vi "calc_rot.vi"(3 "Reference":T1, 4 "Input":T3, 5 "img":u8[][](array[numeric])) -> (0 "Close enough":bool, 1 "angle":dbl, 2 "Output":T2)   [LabVIEW 2024]
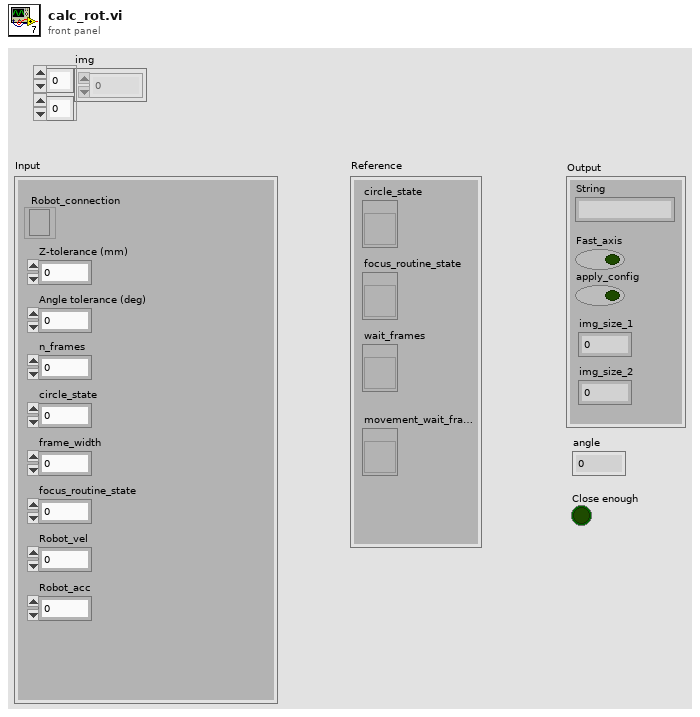
[diagram p1: front panel]
types:
  T1 = cluster{"circle_state":refnum<vi>, "focus_routine_state":refnum<vi>, "wait_frames":refnum<vi>, "movement_wait_frames":refnum<vi>}
  T2 = cluster{"String":string, "Fast_axis":bool, "apply_config":bool, "img_size_1":i32, "img_size_2":i32}
  T3 = cluster{"Robot_connection":refnum<k5>, "Z-tolerance (mm)":dbl, "Angle tolerance (deg)":dbl, "n_frames":i16, "circle_state":i8, "frame_width":i16, "focus_routine_state":i8, "Robot_vel":dbl, "Robot_acc":dbl}
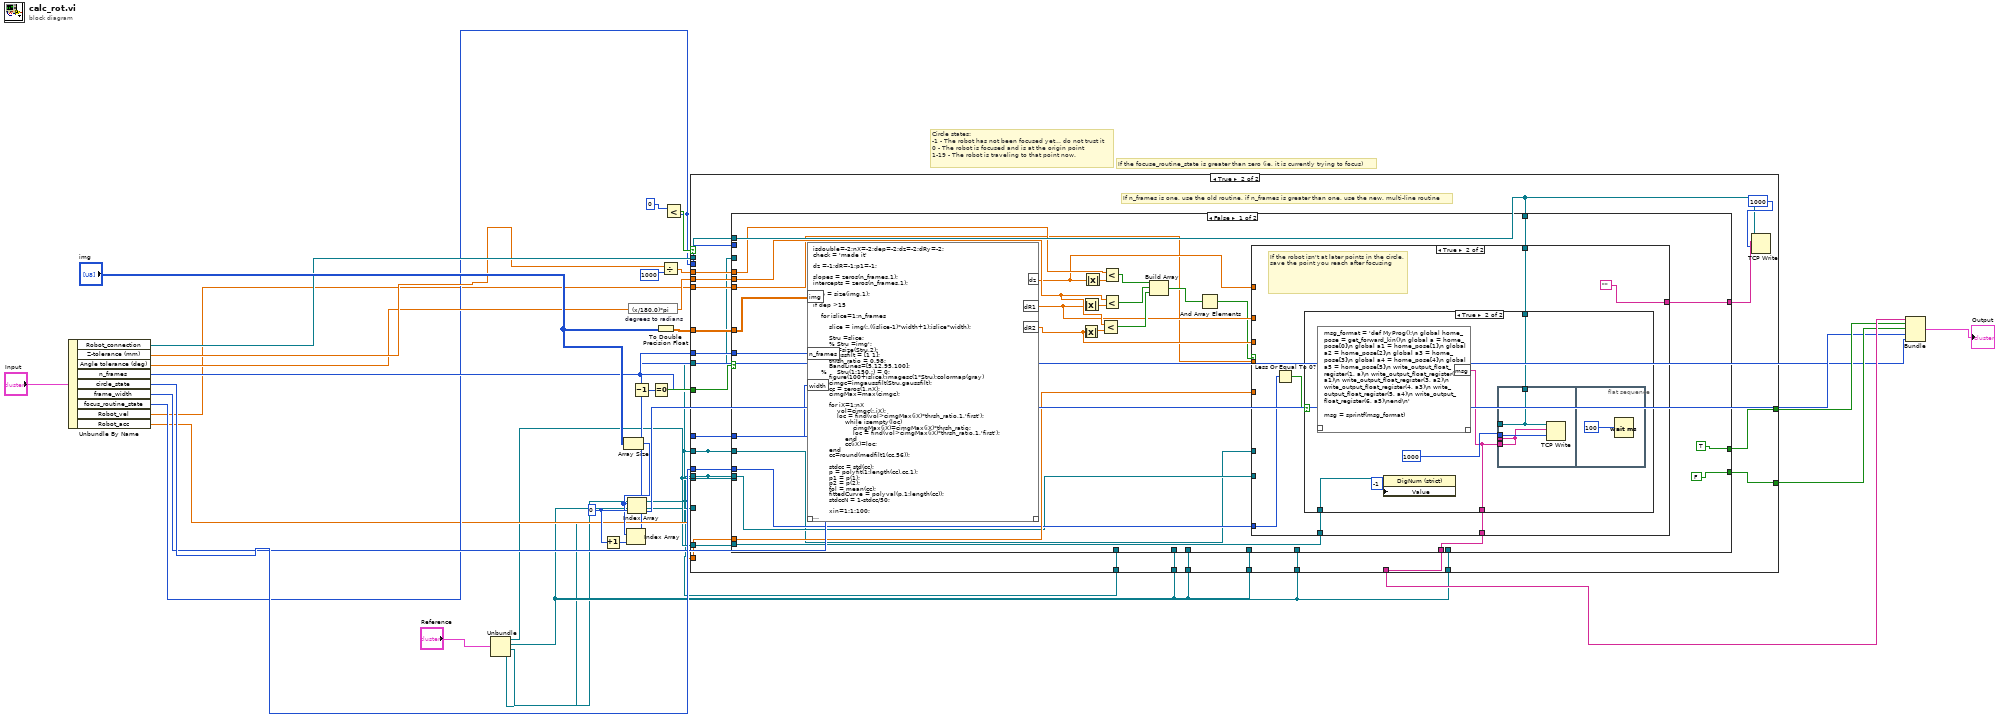
[diagram p0: block diagram]
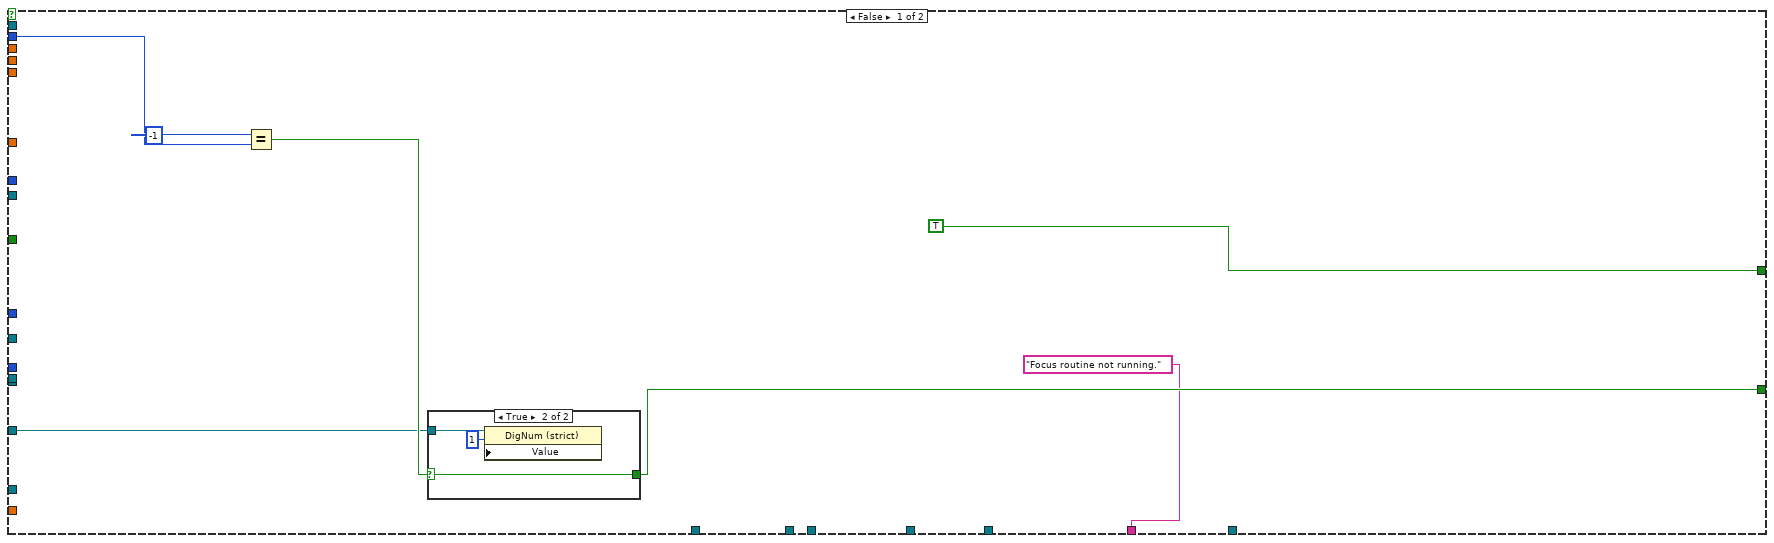
[diagram p2: hidden frame]
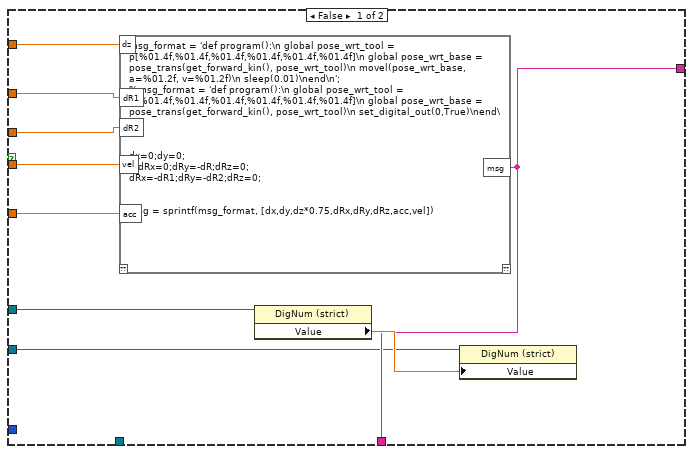
[diagram p4: hidden frame]
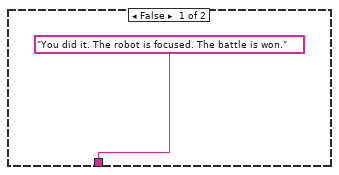
[diagram p5: hidden frame]
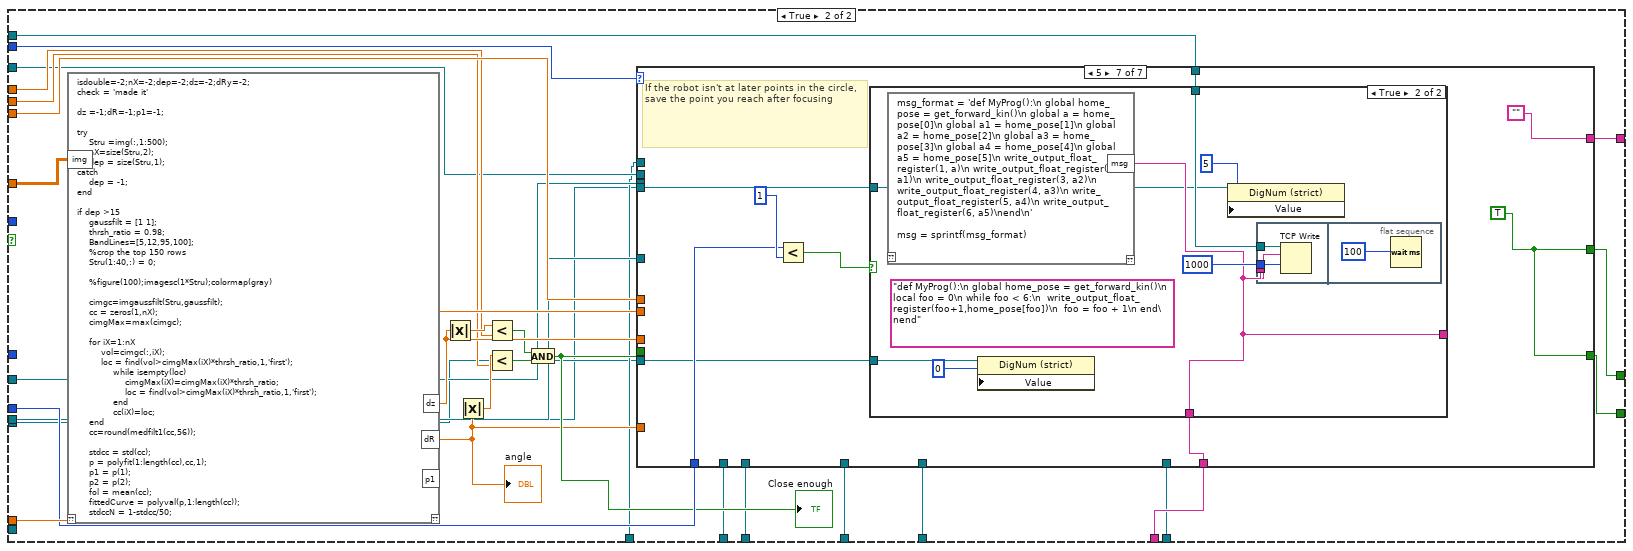
[diagram p6: hidden frame]
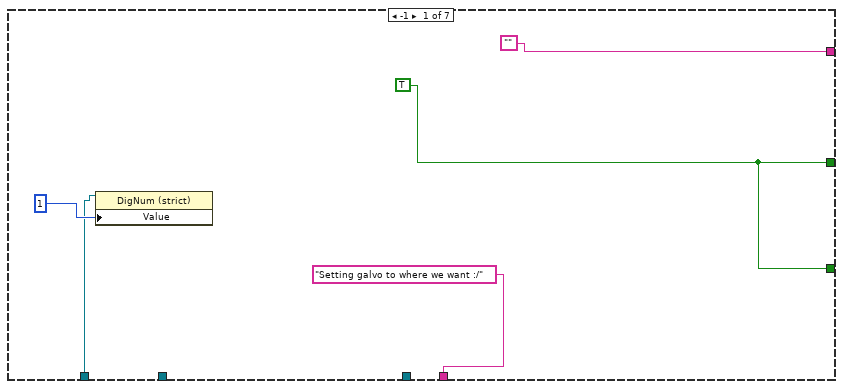
[diagram p7: hidden frame]
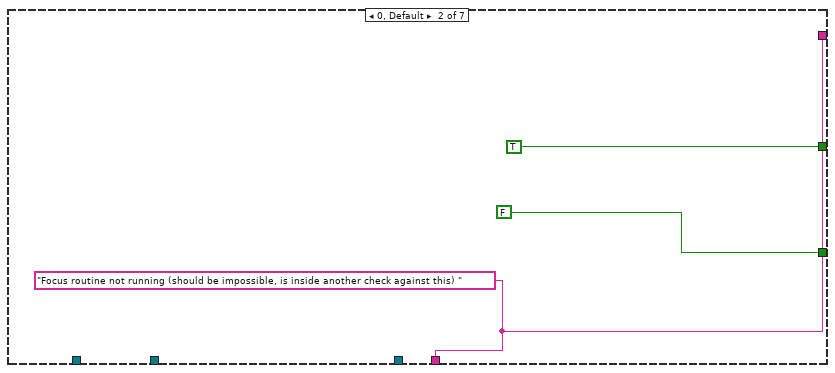
[diagram p8: hidden frame]
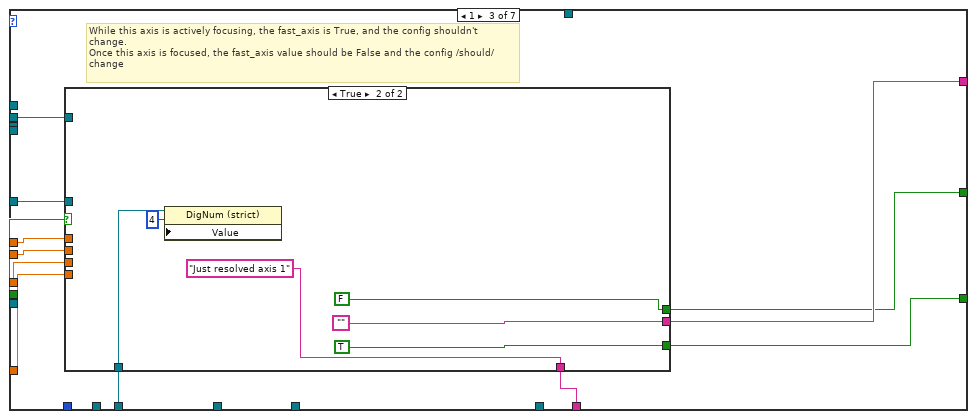
[diagram p9: hidden frame]
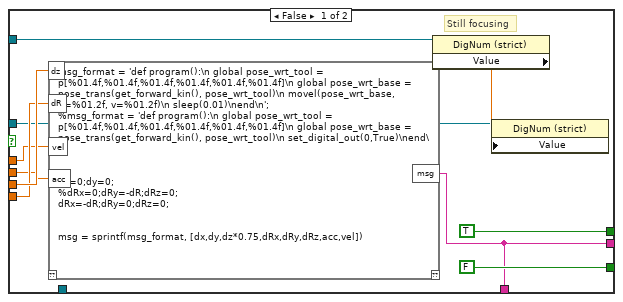
[diagram p10: hidden frame]
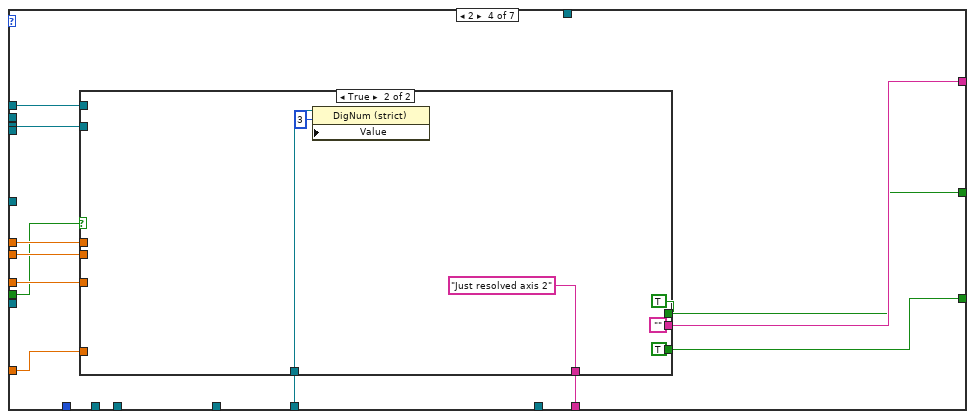
[diagram p11: hidden frame]
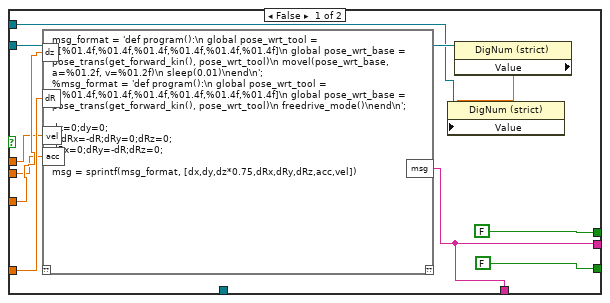
[diagram p12: hidden frame]
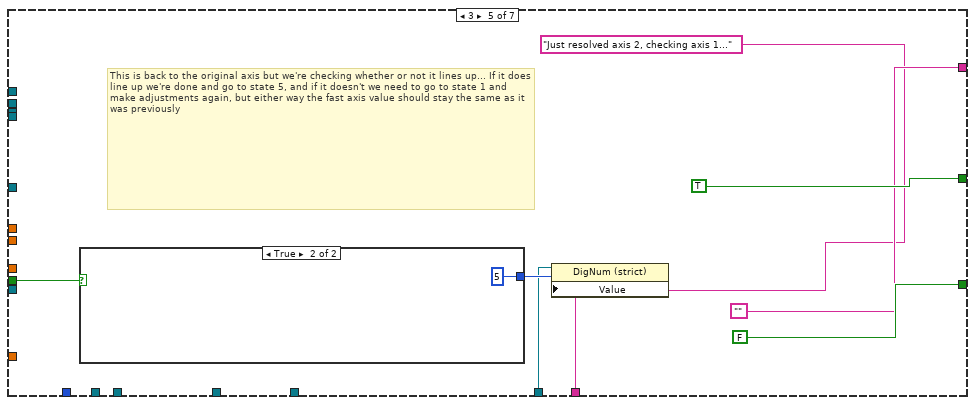
[diagram p13: hidden frame]
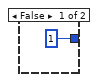
[diagram p14: hidden frame]
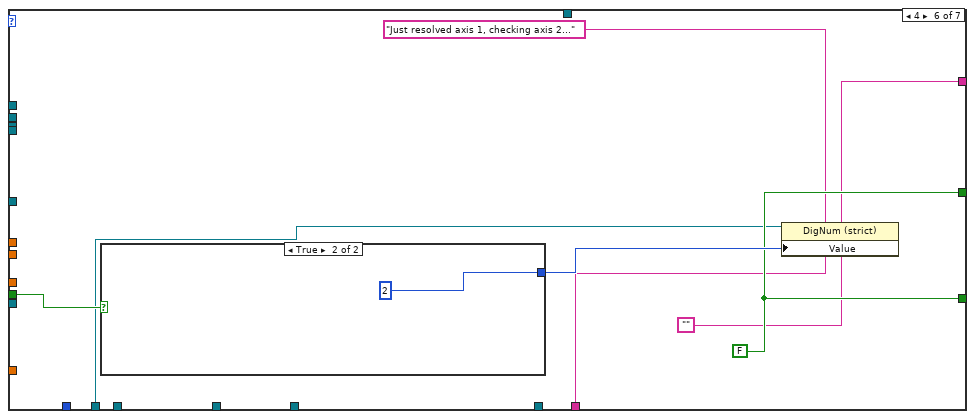
[diagram p15: hidden frame]
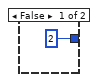
[diagram p16: hidden frame]
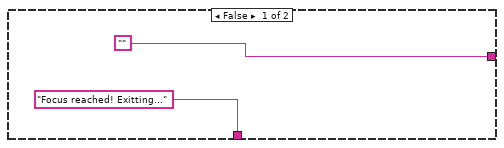
[diagram p17: hidden frame]
diagram:
  w33 = 0
  # "If the focuse_routine_state is greater than zero (ie, it is currently trying to focus)"
  # "Circle states:\n-1 - The robot has not been focused yet... do not trust it\n0 - The robot is focused and is at the origin point\n1-19 - The robot is traveling to that point now."
  n1 = Unbundle By Name("Input") -> ("Robot_connection"=w20:refnum<k5>, "Z-tolerance (mm)"=w19:dbl, "Angle tolerance (deg)"=w18:dbl, "n_frames"=w17:i16, "circle_state"=w16:i8, "frame_width"=w15:i16, "focus_routine_state"=w14:i8, "Robot_vel"=w13:dbl, "Robot_acc"=w12:dbl)
  n2 = Unbundle("Reference") -> ("circle_state"=w4:refnum<vi>, "focus_routine_state"=w3:refnum<vi>, "wait_frames"=w2:refnum<vi>, "movement_wait_frames"=w1:refnum<vi>)
  n3 = Increment(x=w33) -> (x+1=w32:i32)
  n4 = Array Size(array="img") -> (size(s)=w31:i32[])
  n5 = Index Array(array=w31, index=w32) -> (element=w6:i32)
  n6 = Index Array(array=w31, index=w33) -> (element=w7:i32)
  n7 = expression code="(x/180.0)*pi" "degrees to radians"(w18) -> (w25:dbl)
  n8 = Decrement(x=w17) -> (x-1=w28:i16)
  n9 = Equal To 0?(x=w28) -> (x = 0?=w29:bool)
  n10 = To Double Precision Float(number="img") -> (double precision float=w22:dbl[][])
  n11 = Divide(x=w19, y=1000) -> (x/y=w27:dbl)
  n12 = Less?(x=0, y=w14) -> (x < y?=w24:bool)
  n13 = case shown="True" w24 {
    tunnel: w22 -> [_ w71]
    tunnel: w14 -> [w39 w70]
    tunnel: w13 -> [_ w69]
    tunnel: w12 -> [_ w68]
    tunnel: w27 -> [_ w67]
    tunnel: w25 -> [_ w66]
    tunnel: w20 -> [_ w56]
    tunnel: [TRUE w63] -> w9
    tunnel: [w36 w62] -> w8
    tunnel: ["Focus routine not running." w61] -> w10
    tunnel: w16 -> [_ w60]
    tunnel: w29 -> [_ w59]
    tunnel: w15 -> [_ w58]
    tunnel: w17 -> [_ w57]
    tunnel: w3 -> [w34 _]
    tunnel: w4 -> [_ w55]
    tunnel: w3 -> [_ w54]
    tunnel: w1 -> [_ w53]
    tunnel: w3 -> [_ w52]
    tunnel: w1 -> [_ w51]
    tunnel: w2 -> [_ w50]
    tunnel: w3 -> [_ w49]
    tunnel: w3 -> [_ w48]
    tunnel: w3 -> [_ w47]
    tunnel: w4 -> [_ w46]
    tunnel: w2 -> [_ w45]
    frame False {
      n14 = Equal?(x=-1, y=w39) -> (x = y?=w38:bool)
      n15 = case shown="True" w38 {
        selector: w38 -> [w41 w44]
        tunnel: [w41 w44] -> w36
        tunnel: w34 -> [_ w42]
        frame False {
        }
        frame True {
          n16 = property class="DigNum (strict)"(reference=w42, "Value"=1) -> ()  [unwired: 1 in, 2 out]
        }
      }
    }
    frame True {
      # "If n_frames is one, use the old routine, if n_frames is greater than one, use the new, multi-line routine"
      n17 = case shown="False" w59 {
        tunnel: w71 -> [w98 w153]
        tunnel: w70 -> [_ w152]
        tunnel: w69 -> [w82 w151]
        tunnel: w68 -> [w83 w150]
        tunnel: w67 -> [w94 w146]
        tunnel: w66 -> [w90 w145]
        tunnel: [w78 w142] -> w65
        tunnel: [TRUE w141] -> w63
        tunnel: [FALSE w140] -> w62
        tunnel: [w75 w139] -> w61
        tunnel: w60 -> [w76 w138]
        tunnel: w56 -> [_ w136]
        tunnel: w58 -> [w97 _]
        tunnel: w57 -> [w96 _]
        tunnel: w56 -> [w77 _]
        tunnel: w45 -> [w74 _]
        tunnel: w51 -> [w73 _]
        tunnel: w55 -> [w72 _]
        tunnel: w54 -> [_ w134]
        tunnel: w45 -> [_ w133]
        tunnel: w53 -> [_ w132]
        tunnel: w52 -> [_ w131]
        tunnel: w51 -> [_ w130]
        tunnel: w50 -> [_ w129]
        tunnel: w49 -> [_ w128]
        tunnel: w48 -> [_ w127]
        tunnel: w47 -> [_ w126]
        tunnel: w46 -> [_ w125]
        tunnel: w45 -> [_ w124]
        frame False {
          n18 = script code="isdouble=-2;nX=-2;dep=-2;dz=-2;dRy=-2;\ncheck = 'made it'\n\ndz =-1;dR=-1;p1=-1;\n\nslopes = zeros(n_frames,1);\nintercepts = zeros(n_frames,1);\n\ndep = size(img,1);\n    \nif dep >15\n    \n    for islice=1:n_frames\n\n        slice = img(:,((islice-1)*width+1):islice*width);\n        \n        Stru =slice;\n        % Stru =img';\n        nX=size(Stru,2);\n        gaussfilt = [1 1];\n        thrsh_ratio = 0.98;\n        BandLines=[5,12,95,100];\n    %     Stru(1:150,:) = 0;\n        figure(100+islice);imagesc(1*Stru);colormap(gray)\n        cimgc=imgaussfilt(Stru,gaussfilt);\n        cc = zeros(1,nX);\n        cimgMax=max(cimgc);\n    \n        for iX=1:nX\n            vol=cimgc(:,iX);\n            loc = find(vol>cimgMax(iX)*thrsh_ratio,1,'first');\n                while isempty(loc)\n                    cimgMax(iX)=cimgMax(iX)*thrsh_ratio;\n                    loc = find(vol>cimgMax(iX)*thrsh_ratio,1,'first');\n                end\n                cc(iX)=loc;\n        end\n        cc=round(medfilt1(cc,56));\n    \n        stdcc = std(cc);\n        p = polyfit(1:length(cc),cc,1);\n        p1 = p(1);\n        p2 = p(2);\n        fol = mean(cc);\n        fittedCurve = polyval(p,1:length(cc));\n        stdccN = 1-stdcc/50;\n    \n        xin=1:1:100;\n    \n        hold on; plot(cc, 'r')\n        hold on; plot(fittedCurve, 'b')\n    \n        angle_output = 9.65 * atan(p1);\n        output_2 = fol / 51.2;\n    \n        slope = p1;\n        intercept = fol;\n\n        slopes(islice) = slope;\n        intercepts(islice) = intercept;\n    end\n%\n\nend\n\nr1_slope = mean(slopes);\nr1_intercept = mean(intercepts);\nr2_slope = polyfit(round(linspace(1,500,3)),intercepts,1);\nr2_slope = r2_slope(1);\n\n\nr1_slope\nr1_intercept\nr2_slope\n\nangle_output = 9.65 * atan(p1);\noutput_2 = fol / 51.2;\n\ndz=(r1_intercept-210)/150/1000 * 1.2;\ndR1=atan(r1_slope)*0.9\ndR2=atan(r2_slope)*0.9"("img"=w98, "n_frames"=w96, "width"=w97) -> ("dz"=w86:dbl, "dR1"=w85:dbl, "dR2"=w84:dbl)  [unwired: 1 in, 1 out]
          n19 = Absolute Value(x=w84) -> (abs(x)=w92:dbl)
          n20 = Absolute Value(x=w85) -> (abs(x)=w91:dbl)
          n21 = Absolute Value(x=w86) -> (abs(x)=w95:dbl)
          n22 = Less?(x=w90, y=w92) -> (x < y?=w88:bool)
          n23 = Less?(x=w94, y=w95) -> (x < y?=w93:bool)
          n24 = Less?(x=w90, y=w91) -> (x < y?=w89:bool)
          n25 = Build Array(w93, w89, w88) -> (w87:bool[])
          n26 = And Array Elements(Boolean array=w87) -> (logical AND=w81:bool)
          n27 = case shown="True" w81 {
            tunnel: w86 -> [w107 _]
            tunnel: w85 -> [w106 _]
            tunnel: w84 -> [w105 _]
            tunnel: w83 -> [w104 _]
            tunnel: w82 -> [w103 _]
            tunnel: [w101 ""] -> w78
            tunnel: w77 -> [_ w112]
            tunnel: w76 -> [_ w110]
            tunnel: [w101 w109] -> w75
            tunnel: w74 -> [w100 _]
            tunnel: w73 -> [w99 _]
            tunnel: w72 -> [_ w108]
            frame False {
              n28 = script code="msg_format = 'def program():\\n global pose_wrt_tool = p[%01.4f,%01.4f,%01.4f,%01.4f,%01.4f,%01.4f]\\n global pose_wrt_base = pose_trans(get_forward_kin(), pose_wrt_tool)\\n movel(pose_wrt_base, a=%01.2f, v=%01.2f)\\n sleep(0.01)\\nend\\n';\n%msg_format = 'def program():\\n global pose_wrt_tool = p[%01.4f,%01.4f,%01.4f,%01.4f,%01.4f,%01.4f]\\n global pose_wrt_base = pose_trans(get_forward_kin(), pose_wrt_tool)\\n set_digital_out(0,True)\\nend\\n';\n\n\ndx=0;dy=0;\n%dRx=0;dRy=-dR;dRz=0;\ndRx=-dR1;dRy=-dR2;dRz=0;\n\n\nmsg = sprintf(msg_format, [dx,dy,dz*0.75,dRx,dRy,dRz,acc,vel])"("dz"=w107, "dR1"=w106, "vel"=w103, "acc"=w104, "dR2"=w105) -> ("msg"=w101:string)  [unwired: 1 in, 1 out]
              n29 = property class="DigNum (strict)"(reference=w99) -> ("Value"=w102:dbl)  [unwired: 1 in, 2 out]
              n30 = property class="DigNum (strict)"(reference=w100, "Value"=w102) -> ()  [unwired: 1 in, 2 out]
            }
            frame True {
              # "If the robot isn't at later points in the circle, save the point you reach after focusing"
              n31 = Less Or Equal To 0?(x=w110) -> (x <= 0?=w111:bool)
              n32 = case shown="True" w111 {
                tunnel: w112 -> [_ w119]
                tunnel: ["You did it. The robot is focused. The battle is won." w116] -> w109
                tunnel: w108 -> [_ w115]
                frame False {
                }
                frame True {
                  n33 = script code="msg_format = 'def MyProg():\\n global home_pose = get_forward_kin()\\n global a = home_pose[0]\\n global a1 = home_pose[1]\\n global a2 = home_pose[2]\\n global a3 = home_pose[3]\\n global a4 = home_pose[4]\\n global a5 = home_pose[5]\\n write_output_float_register(1, a)\\n write_output_float_register(2, a1)\\n write_output_float_register(3, a2)\\n write_output_float_register(4, a3)\\n write_output_float_register(5, a4)\\n write_output_float_register(6, a5)\\nend\\n'\n\nmsg = sprintf(msg_format)"() -> ("msg"=w116:string)  [unwired: 1 in, 1 out]
                  n34 = property class="DigNum (strict)"(reference=w115, "Value"=-1) -> ()  [unwired: 1 in, 2 out]
                  n35 = flat-sequence {
                    tunnel: [w120] -> _
                    tunnel: [w121] -> _
                    tunnel: 1000 -> [w122]
                    tunnel: w116 -> [w121]
                    tunnel: w119 -> [w120]
                    frame #0 {
                      n36 = TCP Write(connection ID=w120, data in=w121, 9:w122) -> ()  [unwired: 1 in, 3 out]
                    }
                    frame #1 {
                      n37 = Wait (ms)(milliseconds to wait=100) -> ()  [unwired: 1 out]
                    }
                  }
                }
              }
            }
          }
        }
        frame True {
          n38 = script code="isdouble=-2;nX=-2;dep=-2;dz=-2;dRy=-2;\ncheck = 'made it'\n\ndz =-1;dR=-1;p1=-1;\n\ntry\n    Stru =img(:,1:500);\n    nX=size(Stru,2);\n    dep = size(Stru,1);\ncatch\n    dep = -1;\nend\n    \nif dep >15\n    gaussfilt = [1 1];\n    thrsh_ratio = 0.98;\n    BandLines=[5,12,95,100];\n    %crop the top 150 rows\n    Stru(1:40,:) = 0;\n\n    %figure(100);imagesc(1*Stru);colormap(gray)\n    \n    cimgc=imgaussfilt(Stru,gaussfilt);\n    cc = zeros(1,nX);\n    cimgMax=max(cimgc);\n\n    for iX=1:nX\n        vol=cimgc(:,iX);\n        loc = find(vol>cimgMax(iX)*thrsh_ratio,1,'first');\n            while isempty(loc)\n                cimgMax(iX)=cimgMax(iX)*thrsh_ratio;\n                loc = find(vol>cimgMax(iX)*thrsh_ratio,1,'first');\n            end\n            cc(iX)=loc;\n    end\n    cc=round(medfilt1(cc,56));\n\n    stdcc = std(cc);\n    p = polyfit(1:length(cc),cc,1);\n    p1 = p(1);\n    p2 = p(2);\n    fol = mean(cc);\n    fittedCurve = polyval(p,1:length(cc));\n    stdccN = 1-stdcc/50;\n\n    xin=1:1:100;\n\n    %hold on; plot(cc, 'r')\n    %hold on; plot(fittedCurve, 'b')\n\n    angle_output = 9.65 * atan(p1);\n    output_2 = fol / 51.2;\n    dx=0;dy=0;dz=(fol-210)/150/1000 * 1.2;\n    %dRx=0;dRy=atan(p1)*0.2913;dRz=0;\n    dR=atan(p1)*0.9\n% \nend"("img"=w153) -> ("dz"=w149:dbl, "dR"=w135:dbl)  [unwired: 1 in, 2 out]
          "angle" <- w135
          n39 = Absolute Value(x=w149) -> (abs(x)=w147:dbl)
          n40 = Absolute Value(x=w135) -> (abs(x)=w148:dbl)
          n41 = Less?(x=w147, y=w146) -> (x < y?=w144:bool)
          n42 = Less?(x=w148, y=w145) -> (x < y?=w143:bool)
          n43 = And(x=w144, y=w143) -> (x .and. y?=w137:bool)
          "Close enough" <- w137
          n44 = case shown="5" w152 {
            tunnel: w149 -> [_ _ w173 w201 _ _ _]
            tunnel: w135 -> [_ _ w172 w200 _ _ _]
            tunnel: w151 -> [_ _ w171 w198 _ _ _]
            tunnel: w150 -> [_ _ w170 w199 _ _ _]
            tunnel: w137 -> [_ _ w169 w196 w224 w230 _]
            tunnel: ["" w160 w168 w197 "" "" ""] -> w142
            tunnel: [w158 TRUE w166 w194 TRUE w231 w243] -> w141
            tunnel: [w158 FALSE w167 w195 FALSE w231 w243] -> w140
            tunnel: ["Setting galvo to where we want :/" w160 w165 w193 "Just resolved axis 2, checking axis 1..." "Just resolved axis 1, checking axis 2..." w239] -> w139
            tunnel: w138 -> [_ _ _ _ _ _ w241]
            tunnel: w136 -> [_ _ _ _ _ _ w237]
            tunnel: w134 -> [w154 _ _ _ _ _ _]
            tunnel: w133 -> [_ _ w164 _ _ _ _]
            tunnel: w132 -> [_ _ w163 _ _ _ _]
            tunnel: w131 -> [_ _ w162 _ _ _ _]
            tunnel: w130 -> [_ _ _ w192 _ _ _]
            tunnel: w129 -> [_ _ _ w191 _ _ _]
            tunnel: w128 -> [_ _ _ w190 _ _ _]
            tunnel: w127 -> [_ _ _ _ w218 _ _]
            tunnel: w126 -> [_ _ _ _ _ w227 _]
            tunnel: w125 -> [_ _ _ _ _ _ w236]
            tunnel: w124 -> [_ _ _ _ _ _ w235]
            frame -1 {
              w158 = TRUE
              n45 = property class="DigNum (strict)"(reference=w154, "Value"=1) -> ()  [unwired: 1 in, 2 out]
            }
            frame 0, Default {
              w160 = "Focus routine not running (should be impossible, is inside another check against this) "
            }
            frame 1 {
              # "While this axis is actively focusing, the fast_axis is True, and the config shouldn't change.\nOnce this axis is focused, the fast_axis value should be False and the config /should/ change"
              n46 = case shown="True" w169 {
                tunnel: w173 -> [w183 _]
                tunnel: w172 -> [w182 _]
                tunnel: w171 -> [w181 _]
                tunnel: w170 -> [w180 _]
                tunnel: [w177 ""] -> w168
                tunnel: [FALSE TRUE] -> w167
                tunnel: [TRUE FALSE] -> w166
                tunnel: [w177 "Just resolved axis 1"] -> w165
                tunnel: w164 -> [w175 _]
                tunnel: w163 -> [w174 _]
                tunnel: w162 -> [_ w184]
                frame False {
                  # "Still focusing"
                  n47 = script code="msg_format = 'def program():\\n global pose_wrt_tool = p[%01.4f,%01.4f,%01.4f,%01.4f,%01.4f,%01.4f]\\n global pose_wrt_base = pose_trans(get_forward_kin(), pose_wrt_tool)\\n movel(pose_wrt_base, a=%01.2f, v=%01.2f)\\n sleep(0.01)\\nend\\n';\n%msg_format = 'def program():\\n global pose_wrt_tool = p[%01.4f,%01.4f,%01.4f,%01.4f,%01.4f,%01.4f]\\n global pose_wrt_base = pose_trans(get_forward_kin(), pose_wrt_tool)\\n set_digital_out(0,True)\\nend\\n';\n\n\ndx=0;dy=0;\n%dRx=0;dRy=-dR;dRz=0;\ndRx=-dR;dRy=0;dRz=0;\n\n\nmsg = sprintf(msg_format, [dx,dy,dz*0.75,dRx,dRy,dRz,acc,vel])"("dz"=w183, "dR"=w182, "vel"=w181, "acc"=w180) -> ("msg"=w177:string)  [unwired: 1 in, 1 out]
                  n48 = property class="DigNum (strict)"(reference=w174) -> ("Value"=w176:dbl)  [unwired: 1 in, 2 out]
                  n49 = property class="DigNum (strict)"(reference=w175, "Value"=w176) -> ()  [unwired: 1 in, 2 out]
                }
                frame True {
                  n50 = property class="DigNum (strict)"(reference=w184, "Value"=4) -> ()  [unwired: 1 in, 2 out]
                }
              }
            }
            frame 2 {
              # "While this axis is actively focusing, the fast_axis is False, and the config shouldn't change.\nOnce this axis is focused, the fast_axis value should be True and the config /should/ change"
              n51 = case shown="True" w196 {
                tunnel: w201 -> [w211 _]
                tunnel: w200 -> [w210 _]
                tunnel: w199 -> [w209 _]
                tunnel: w198 -> [w208 _]
                tunnel: [w205 ""] -> w197
                tunnel: [FALSE TRUE] -> w195
                tunnel: [FALSE TRUE] -> w194
                tunnel: [w205 "Just resolved axis 2"] -> w193
                tunnel: w192 -> [w203 _]
                tunnel: w191 -> [w202 _]
                tunnel: w190 -> [_ w212]
                frame False {
                  n52 = script code="msg_format = 'def program():\\n global pose_wrt_tool = p[%01.4f,%01.4f,%01.4f,%01.4f,%01.4f,%01.4f]\\n global pose_wrt_base = pose_trans(get_forward_kin(), pose_wrt_tool)\\n movel(pose_wrt_base, a=%01.2f, v=%01.2f)\\n sleep(0.01)\\nend\\n';\n%msg_format = 'def program():\\n global pose_wrt_tool = p[%01.4f,%01.4f,%01.4f,%01.4f,%01.4f,%01.4f]\\n global pose_wrt_base = pose_trans(get_forward_kin(), pose_wrt_tool)\\n freedrive_mode()\\nend\\n';\n\ndx=0;dy=0;\n%dRx=-dR;dRy=0;dRz=0;\ndRx=0;dRy=-dR;dRz=0;\n\nmsg = sprintf(msg_format, [dx,dy,dz*0.75,dRx,dRy,dRz,acc,vel])"("dz"=w211, "dR"=w210, "acc"=w209, "vel"=w208) -> ("msg"=w205:string)  [unwired: 1 in, 1 out]
                  n53 = property class="DigNum (strict)"(reference=w203) -> ("Value"=w204:dbl)  [unwired: 1 in, 2 out]
                  n54 = property class="DigNum (strict)"(reference=w202, "Value"=w204) -> ()  [unwired: 1 in, 2 out]
                }
                frame True {
                  n55 = property class="DigNum (strict)"(reference=w212, "Value"=3) -> ()  [unwired: 1 in, 2 out]
                }
              }
            }
            frame 3 {
              # "This is back to the original axis but we're checking whether or not it lines up... If it does line up we're done and go to state 5, and if it doesn't we need to go to state 1 and make adjustments again, but either way the fast axis value should stay the same as it was previously"
              n56 = case shown="True" w224 {
                tunnel: [1 5] -> w223
                frame False {
                }
                frame True {
                }
              }
              n57 = property class="DigNum (strict)"(reference=w218, "Value"=w223) -> ()  [unwired: 1 in, 2 out]
            }
            frame 4 {
              w231 = FALSE
              n58 = case shown="True" w230 {
                tunnel: [2 2] -> w232
                frame False {
                }
                frame True {
                }
              }
              n59 = property class="DigNum (strict)"(reference=w227, "Value"=w232) -> ()  [unwired: 1 in, 2 out]
            }
            frame 5 {
              w243 = TRUE
              # "If the robot isn't at later points in the circle, save the point you reach after focusing"
              n60 = Less?(x=w241, y=1) -> (x < y?=w240:bool)
              n61 = case shown="True" w240 {
                tunnel: ["" w248] -> _
                tunnel: ["Focus reached! Exitting..." w248] -> w239
                tunnel: w237 -> [_ w250]
                tunnel: w236 -> [_ w247]
                tunnel: w235 -> [_ w246]
                frame False {
                }
                frame True {
                  (unwired) "def MyProg():\n global home_pose = get_forward_kin()\n local foo = 0\n while foo < 6:\n  write_output_float_register(foo+1,home_pose[foo])\n  foo = foo + 1\n end\nend"
                  n62 = script code="msg_format = 'def MyProg():\\n global home_pose = get_forward_kin()\\n global a = home_pose[0]\\n global a1 = home_pose[1]\\n global a2 = home_pose[2]\\n global a3 = home_pose[3]\\n global a4 = home_pose[4]\\n global a5 = home_pose[5]\\n write_output_float_register(1, a)\\n write_output_float_register(2, a1)\\n write_output_float_register(3, a2)\\n write_output_float_register(4, a3)\\n write_output_float_register(5, a4)\\n write_output_float_register(6, a5)\\nend\\n'\n\nmsg = sprintf(msg_format)"() -> ("msg"=w248:string)  [unwired: 1 in, 1 out]
                  n63 = property class="DigNum (strict)"(reference=w247, "Value"=0) -> ()  [unwired: 1 in, 2 out]
                  n64 = property class="DigNum (strict)"(reference=w246, "Value"=5) -> ()  [unwired: 1 in, 2 out]
                  n65 = flat-sequence {
                    tunnel: w250 -> [w255]
                    tunnel: w248 -> [w254]
                    tunnel: 1000 -> [w253]
                    frame #0 {
                      n66 = TCP Write(connection ID=w255, data in=w254, 9:w253) -> ()  [unwired: 1 in, 3 out]
                    }
                    frame #1 {
                      n67 = Wait (ms)(milliseconds to wait=100) -> ()  [unwired: 1 out]
                    }
                  }
                }
              }
            }
          }
        }
      }
      n68 = TCP Write(connection ID=w56, data in=w65, 9:1000) -> ()  [unwired: 1 in, 3 out]
    }
  }
  n69 = Bundle(w10, w9, w8, w7, w6) -> (→"Output":cluster{string, bool, bool, i32, i32})  [unwired: 1 in]
